vi "Read.vi"(8 "error in (no error)":errorcluster, 11 "Abs_Variant in":refnum<class "Abs_Variant.lvclass">) -> (0 "error out":errorcluster, 2 "Variant":variant, 3 "Abs_Variant out":refnum<class "Abs_Variant.lvclass">)   [LabVIEW 2021, in "Abs_Variant.lvclass"]
uses:
  Abs_Variant.lvclass
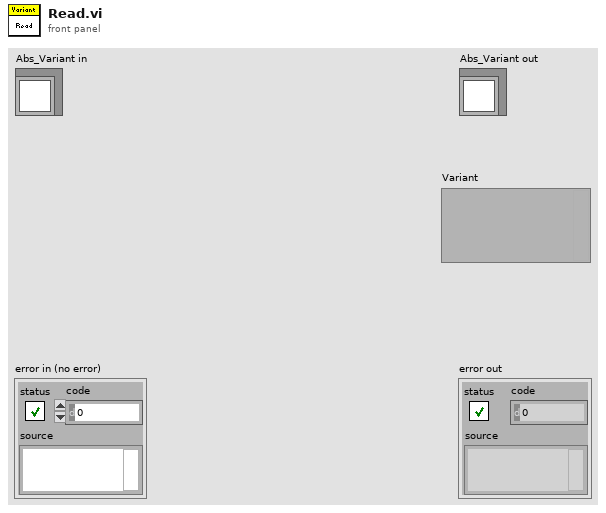
[diagram p1: front panel]
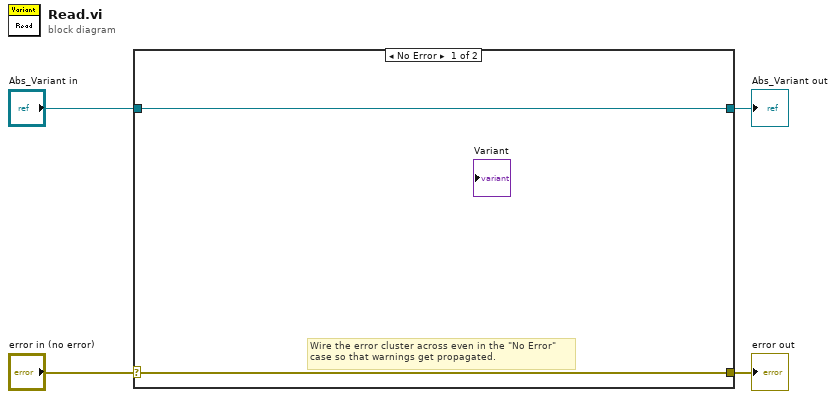
[diagram p0: block diagram]
diagram:
  n1 = case shown="No Error" "error in (no error)" {
    selector: "error in (no error)" -> [w5 w8]
    tunnel: [w5 w8] -> w3
    tunnel: [w6 w7] -> w1
    tunnel: "Abs_Variant in" -> [w6 w7]
    frame No Error {
      # "Wire the error cluster across even in the \"No Error\"\ncase so that warnings get propagated."
    }
    frame Error {
    }
  }
  "error out" <- w3
  "Abs_Variant out" <- w1
